vi "VISA  Send Receive.vi"(1 "RDY max wait, ms (-1 = forever)":i32=500, 4 "RDY when up":bool=TRUE, 5 "Data ready bit (-1 - ignore)":i32=-1, 6 "Read terminator":i16, 7 "Read Delay, ms":u32, 8 "error in (no error)":errorcluster, 9 "Receive count":i32=256, 10 "data string in":string, 11 "VISA Resource Name":refnum<visa-resource-name>) -> (0 "error out":errorcluster, 2 "data string out":string, 3 "VISA Resource Name Out":refnum<visa-resource-name>)   [LabVIEW 2021]
panel:
  out "data string in":string
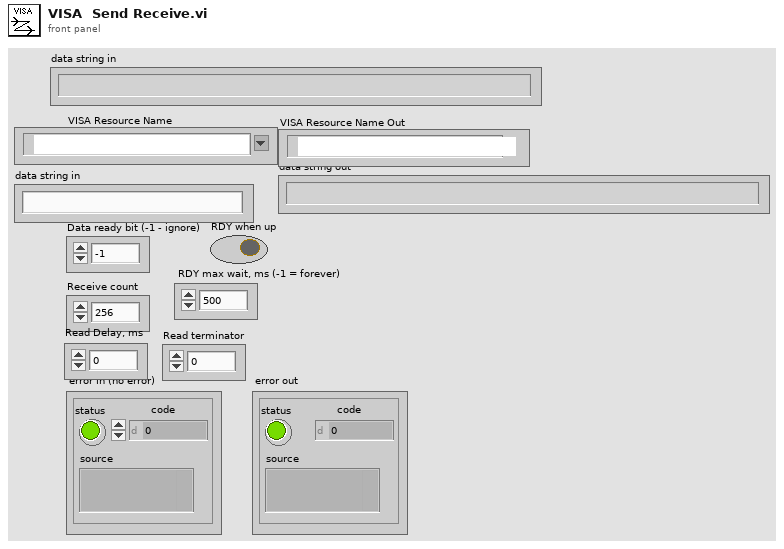
[diagram p1: front panel]
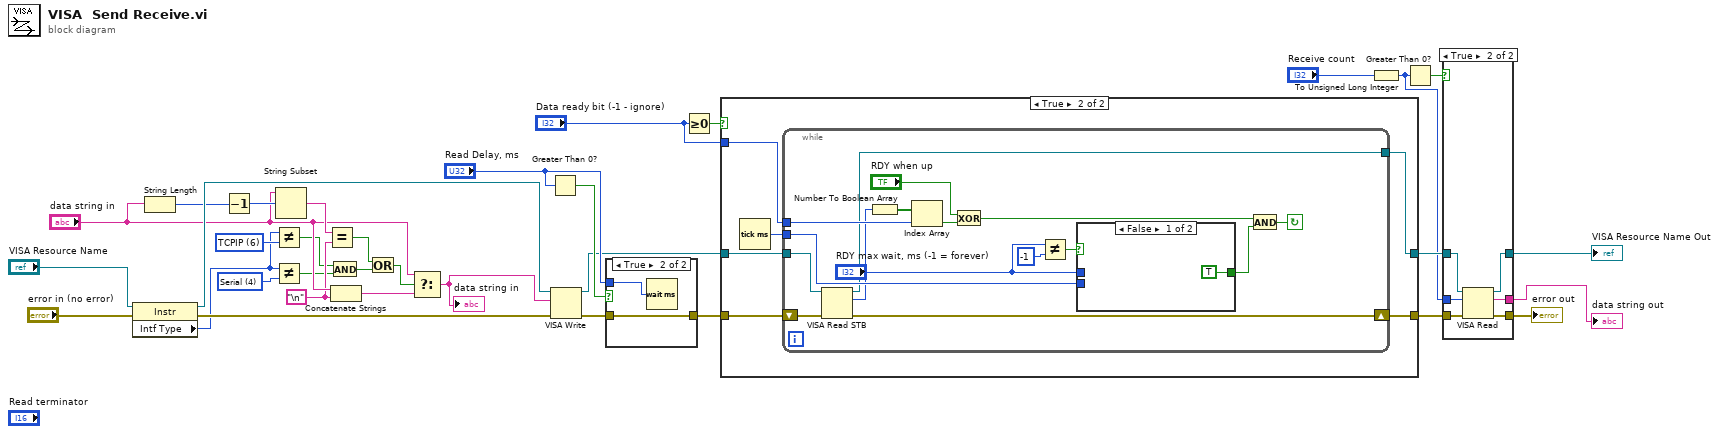
[diagram p0: block diagram]
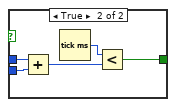
[diagram p4: hidden frame]
diagram:
  w5 = u16 4 items=["GPIB"=1, "VXI"=2, "GPIB-VXI"=3, "Serial"=4, "PXI"=5, "TCPIP"=6, "USB"=7, "FireWire"=9] ("Interface Information:Interface Type")
  w12 = "\n"
  w17 = u16 6 items=["GPIB"=1, "VXI"=2, "GPIB-VXI"=3, "Serial"=4, "PXI"=5, "TCPIP"=6, "USB"=7, "FireWire"=9] ("Interface Information:Interface Type")
  n1 = property class="Instr"(reference="VISA Resource Name", error in="error in (no error)") -> (reference out=w18:refnum<visa-resource-name>, error out=w20:errorcluster, "Intf Type"=w4:u16)
  n2 = String Length(string="data string in") -> (length=w16:i32)
  n3 = Decrement(x=w16) -> (x-1=w15:i32)
  n4 = Not Equal?(x=w4, y=w17) -> (x != y?=w3:bool)
  n5 = Not Equal?(x=w4, y=w5) -> (x != y?=w2:bool)
  n6 = String Subset(string="data string in", offset (0)=w15) -> (substring=w14:string)  [unwired: 1 in]
  n7 = Equal?(x=w14, y=w12) -> (x = y?=w9:bool)
  n8 = And(x=w3, y=w2) -> (x .and. y?=w1:bool)
  n9 = Concatenate Strings("data string in", w12) -> (w11:string)
  n10 = Or(x=w9, y=w1) -> (x .or. y?=w10:bool)
  n11 = Select(t="data string in", s=w10, f=w11) -> (s? t:f=w6:string)
  "data string in" <- w6
  n12 = Greater Than 0?(x="Read Delay, ms") -> (x > 0?=w32:bool)
  n13 = VISA Write(VISA resource name=w18, write buffer=w6, error in (no error)=w20) -> (VISA resource name out=w25:refnum<visa-resource-name>, error out=w31:errorcluster)  [unwired: 1 out]
  n14 = case shown="True" w32 {
    tunnel: w31 -> [w35 w36]
    tunnel: [w35 w36] -> w28
    tunnel: "Read Delay, ms" -> [_ w37]
    frame False {
    }
    frame True {
      n15 = Wait (ms)(milliseconds to wait=w37) -> ()  [unwired: 1 out]
    }
  }
  n16 = Greater Or Equal To 0?(x="Data ready bit (-1 - ignore)") -> (x >= 0?=w29:bool)
  n17 = case shown="True" w29 {
    tunnel: w28 -> [w39 w44]
    tunnel: "Data ready bit (-1 - ignore)" -> [_ w43]
    tunnel: [w39 w42] -> w26
    tunnel: w25 -> [w38 w41]
    tunnel: [w38 w40] -> w24
    frame False {
    }
    frame True {
      n18 = Tick Count (ms)() -> (millisecond timer value=w45:u32)
      n19 = while {
        shift-right: [w60] -> w42
        shift-left: w44 -> [w61]
        tunnel: w45 -> [w57]
        tunnel: w43 -> [w55]
        tunnel: w41 -> [w51]
        tunnel: [w49] -> w40
        stop <- w59 continue-if-true
        n20 = VISA Read STB(8:w61, 11:w51) -> (0:w60:errorcluster, 2:w50:u16, 3:w49:refnum<visa-resource-name>)
        n21 = Number To Boolean Array(number=w50) -> (Boolean array=w56:bool[])
        n22 = Index Array(array=w56, index=w55) -> (element=w54:bool)
        n23 = Exclusive Or(1:w54, 2:"RDY when up") -> (0:w53:bool)
        n24 = Not Equal?(x="RDY max wait, ms (-1 = forever)", y=-1) -> (x != y?=w48:bool)
        n25 = case shown="False" w48 {
          tunnel: [TRUE w67] -> w58
          tunnel: w57 -> [_ w65]
          tunnel: "RDY max wait, ms (-1 = forever)" -> [_ w63]
          frame False {
          }
          frame True {
            n26 = Add(x=w63, y=w65) -> (x+y=w66:u32)
            n27 = Tick Count (ms)() -> (millisecond timer value=w64:u32)
            n28 = Less?(x=w64, y=w66) -> (x < y?=w67:bool)
          }
        }
        n29 = And(x=w53, y=w58) -> (x .and. y?=w59:bool)
      }
    }
  }
  n30 = To Unsigned Long Integer(number="Receive count") -> (unsigned 32bit integer=w8:u32)
  n31 = Greater Than 0?(x=w8) -> (x > 0?=w7:bool)
  n32 = case shown="True" w7 {
    tunnel: [w69 w75] -> w33
    tunnel: w26 -> [w69 w74]
    tunnel: w24 -> [w68 w73]
    tunnel: w8 -> [_ w72]
    tunnel: [_ w71] -> w22
    tunnel: [w68 w70] -> w21
    frame False {
    }
    frame True {
      n33 = VISA Read(VISA resource name=w73, byte count=w72, error in (no error)=w74) -> (VISA resource name out=w70:refnum<visa-resource-name>, read buffer=w71:string, error out=w75:errorcluster)  [unwired: 1 out]
    }
  }
  "error out" <- w33
  "data string out" <- w22
  "VISA Resource Name Out" <- w21
